vi "Remove vims from files in directory.vi"(8 "error in (no error)":errorcluster, 11 "Folder Path":path) -> (0 "error out":errorcluster)   [LabVIEW 2020]
uses:
  <vilib>/Utility/miscctls.llb/LVMapReplaceAction.ctl
  <vilib>/Utility/traverseref.llb/TRef TravTarget.ctl
  6b92614a-126e-4e2c-8477-dc2805cc9e45.vi
  c56adb90-e54b-4597-b7fa-d326b7dff2e6.vi
  <vilib>/Utility/traverseref.llb/VI Scripting - Traverse.lvlib
panel:
  out "Deleting .vim from disk":path
  out "Disconnecting .vim from library":path
  out "Scanning VI...":path
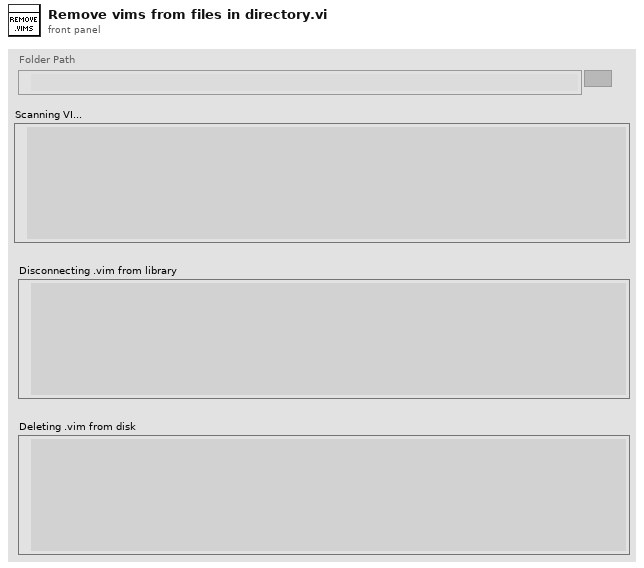
[diagram p1: front panel]
types:
  T1 = enum32{"Invalid", "Standard", "Closed", "Hidden", "Minimized", "Maximized"}
  T2 = typedef "LVMapReplaceAction.ctl" = enum32{"Modify Entry only if found", "Add or Modify Entry", "Delete Entry"}
  T3 = typedef "TRef TravTarget.ctl" = enum16{"FP", "BD", "Other"}
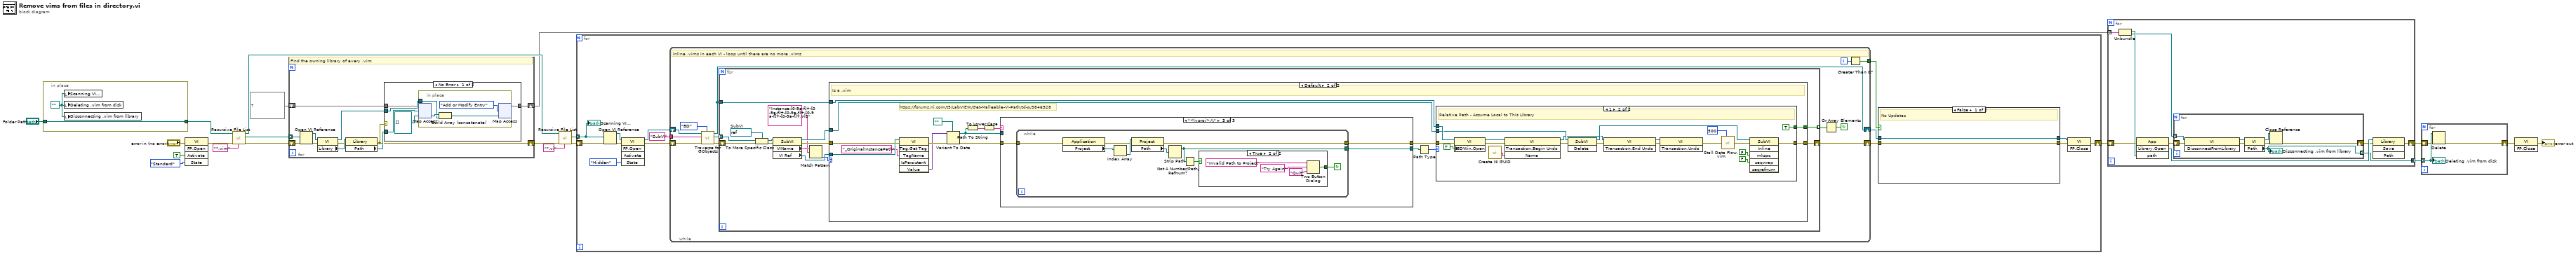
[diagram p0: block diagram]
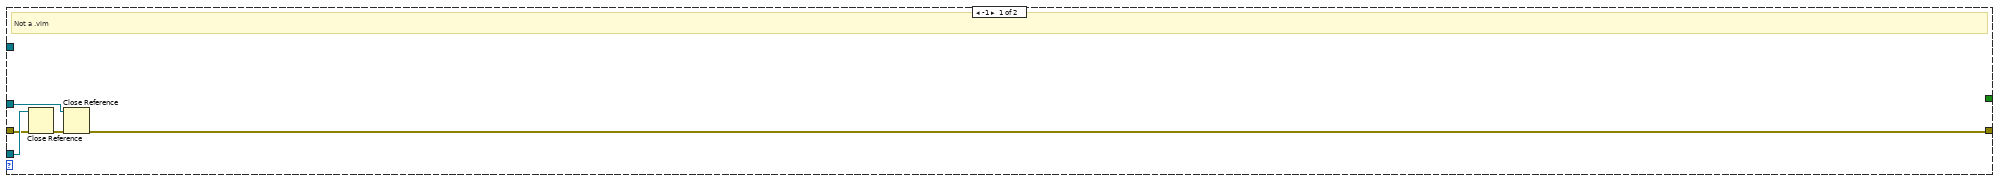
[diagram p2: hidden frame]
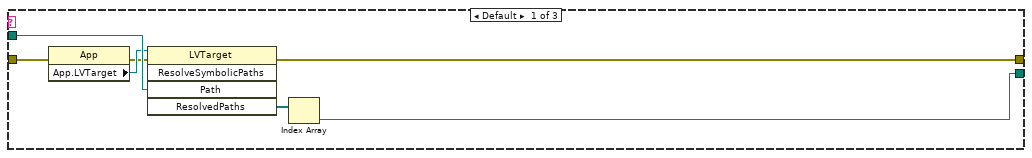
[diagram p3: hidden frame]
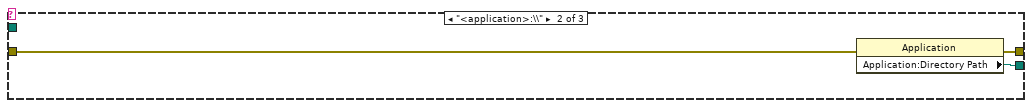
[diagram p4: hidden frame]
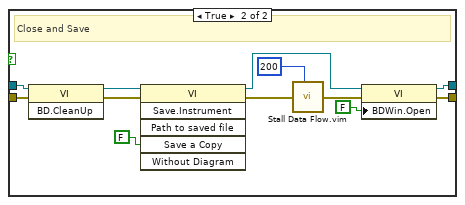
[diagram p7: hidden frame]
diagram:
  n1 = in-place {
    in-place-border: [w22] -> w7
    in-place-border: "Folder Path" -> [w22]
    w23 = path "" ("Scanning VI...")
    n2 = local write "Scanning VI..."(w23) -> ()
    n3 = local write "Deleting .vim from disk"(w23) -> ()
    n4 = local write "Disconnecting .vim from library"(w23) -> ()
  }
  n5 = invoke class="VI" method="FP.Open"(error in="error in (no error)", "Activate"=TRUE ("Activate?"), "State"=T1."Standard") -> (error out=w4:errorcluster)  [unwired: 2 in, 4 out]
  n6 = call <vilib>:"Recursive File List.vi"("pattern"="*.vim", "error in (no error)"=w4, "Folder Path"=w7) -> ("error out"=w19:errorcluster, "All Files in Dir"=w20:path[], "dup Folder Path"=w15:path)  [unwired: 4 in, 2 out]
  n7 = for {
    tunnel: w20 -> [w31] mode=indexing
    shift-right: [w29] -> w11
    shift-left: map{path, refnum<vi>[]} {} ("Size: 0") -> [w28]
    shift-right: [w24] -> w17
    shift-left: w19 -> [w34]
    # "Find the owning library of every .vim"
    n8 = Open VI Reference(vi path=w31, error in (no error)=w34) -> (vi reference=w33:refnum<vi>, error out=w32:errorcluster)  [unwired: 4 in]
    n9 = property class="VI"(reference=w33, error in=w32) -> (reference out=w30:refnum<vi>, error out=w26:errorcluster, "Library"=w27:refnum<vi>)
    n10 = property class="Library"(reference=w27, error in=w26) -> (error out=w24:errorcluster, "Path"=w25:path)  [unwired: 1 out]
    n11 = case shown="No Error" w24 {
      tunnel: w30 -> [w39 _]
      tunnel: [w37 w44] -> w29
      tunnel: w28 -> [w36 w44]
      tunnel: w25 -> [w35 _]
      frame No Error {
        n12 = in-place {
          in-place-border: w39 -> [w41]
          n13 = in-place-map #1(w36, w35, refnum<vi>[] []) -> (w43:refnum<vi>[])  [unwired: 1 out]
          n14 = Build Array (concatenate)(w43, w41) -> (w40:refnum<vi>[])
          n15 = in-place-map #1(w40, LVMapReplaceAction."Add or Modify Entry" ("action")) -> (w37:map{path, refnum<vi>[]})  [unwired: 2 out]
        }
      }
      frame Error {
      }
    }
  }
  n16 = call <vilib>:"Recursive File List.vi"("pattern"="*.vi", "error in (no error)"=w17, "Folder Path"=w15) -> ("error out"=w14:errorcluster, "All Files in Dir"=w13:path[])  [unwired: 4 in, 3 out]
  n17 = for {
    shift-right: [w54] -> w12
    shift-left: w14 -> [w53]
    tunnel: w13 -> [w51] mode=indexing
    n18 = Open VI Reference(vi path=w51, error in (no error)=w53) -> (vi reference=w45:refnum<vi>, error out=w52:errorcluster)  [unwired: 4 in]
    n19 = invoke class="VI" method="FP.Open"(reference=w45, error in=w52, "State"=T1."Hidden") -> (reference out=w55:refnum<vi>, error out=w50:errorcluster)  [unwired: 2 in, 3 out]
    n20 = while {
      shift-right: [w67] -> w48
      shift-left: w55 -> [w68]
      shift-right: [w69] -> w57
      shift-left: w50 -> [w66]
      tunnel: [w60] -> w49
      tunnel: "SubVI" ("Class Name") -> [w59]
      i -> [w61]
      stop <- w62 continue-if-true
      # "Inline .vims in each VI - loop until there are no more .vims"
      n21 = call <vilib>:"Traverse for GObjects.vi"("Traverse Target"=TRef_TravTarget."BD", "error in (no error)"=w66, "Class Name"=w59, "VI Refnum"=w68) -> ("error out"=w65:errorcluster, "References"=w63:refnum<vi>[], "dup VI Refnum"=w67:refnum<vi>)  [unwired: 4 in, 1 out]
      n22 = for {
        shift-right: [w78] -> w69
        shift-left: w65 -> [w84]
        tunnel: w63 -> [w83] mode=indexing
        tunnel: w67 -> [w77]
        tunnel: [w76] -> w70 mode=indexing
        w82 = refnum<vi> refnum  # SubVI
        n23 = To More Specific Class(target class=w82, reference=w83, error in=w84) -> (specific class reference=w81:refnum<vi>, error out=w80:errorcluster)
        n24 = property class="SubVI"(reference=w81, error in=w80) -> (reference out=w72:refnum<vi>, error out=w75:errorcluster, "VIName"=w79:string, "VI Ref"=w73:refnum<vi>)
        n25 = Match Pattern(string=w79, regular expression="Instance:[0-9a-f]+-[0-9a-f]+-[0-9a-f]+-[0-9a-f]+-[0-9a-f]+.vi$") -> (offset past match=w74:i32)  [unwired: 1 in, 3 out]
        n26 = case shown="Default" w74 {
          tunnel: [w89 w106] -> w78
          tunnel: w73 -> [w87 w98]
          tunnel: w77 -> [_ w105]
          tunnel: [_ w104] -> w76
          tunnel: w75 -> [w85 w99]
          tunnel: w72 -> [w88 w103]
          frame -1 {
            # "Not a .vim"
            n27 = Close Reference(reference=w87, error in (no error)=w85) -> (error out=w86:errorcluster)
            n28 = Close Reference(reference=w88, error in (no error)=w86) -> (error out=w89:errorcluster)
          }
          frame Default {
            # "https://forums.ni.com/t5/LabVIEW/Get-Malleable-VI-Path/td-p/3846528"
            # "Is a .vim"
            n29 = invoke class="VI" method="Tag.Get Tag"(reference=w98, error in=w99, "TagName"="_OriginalInstancePath" ("Tag Name")) -> (error out=w102:errorcluster, "Value"=w101:variant)  [unwired: 3 in, 4 out]
            n30 = Variant To Data(error in=w102, type=path "", Variant=w101) -> (data=w94:path, error out=w97:errorcluster)
            n31 = Path To String(path=w94) -> (string=w90:string)
            n32 = To Lower Case(string=w90) -> (all lower case string=w91:string)
            n33 = case shown="\"<lvproj>:\\\\\"" w91 {
              tunnel: w94 -> [w110 _ _]
              tunnel: [w113 w116 w117] -> w93
              tunnel: [w112 w115 w119] -> w95
              tunnel: w97 -> [w111 w114 w118]
              frame Default {
                n34 = property class="App"(error in=w111) -> (error out=w108:errorcluster, "App.LVTarget"=w109:refnum<vi>)  [unwired: 1 in, 1 out]
                n35 = invoke class="LVTarget" method="ResolveSymbolicPaths"(reference=w109, error in=w108, "Path"=w110) -> (error out=w112:errorcluster, "ResolvedPaths"=w107:path[])  [unwired: 2 in, 3 out]
                n36 = Index Array(array=w107) -> (element=w113:path)  [unwired: 1 in]
              }
              frame "<application>:\\" {
                n37 = property class="Application"(error in=w114) -> (error out=w115:errorcluster, "Application:Directory Path"=w116:path)  [unwired: 1 in, 1 out]
              }
              frame "<lvproj>:\\" {
                n38 = while {
                  tunnel: [w125] -> w119
                  tunnel: w118 -> [w124]
                  tunnel: [w121] -> w117
                  stop <- w120 continue-if-true
                  n39 = property class="Application"(error in=w124) -> (error out=w126:errorcluster, "Project"=w128:refnum<vi>[])  [unwired: 1 in, 1 out]
                  n40 = Index Array(array=w128) -> (element=w127:refnum<vi>)  [unwired: 1 in]
                  n41 = property class="Project"(reference=w127, error in=w126) -> (error out=w125:errorcluster, "Path"=w123:path)  [unwired: 1 out]
                  n42 = Strip Path(path=w123) -> (stripped path=w121:path)  [unwired: 1 out]
                  n43 = Not A Number/Path/Refnum?(number/path/refnum=w121) -> (NaN/Path/Refnum?=w122:bool)
                  n44 = case shown="True" w122 {
                    tunnel: [_ w129] -> w120
                    frame False {
                    }
                    frame True {
                      n45 = Two Button Dialog(message="Invalid Path to Project", 1:"Quit" ("F button name (\"Cancel\")"), 2:"Try Again" ("T button name (\"OK\")")) -> (T button?=w129:bool)
                    }
                  }
                }
              }
            }
            n46 = Path Type(1:w93) -> (0:w92:i16)
            n47 = case shown="1" w92 {
              tunnel: w105 -> [_ w153]
              tunnel: [w133 w152] -> w106
              tunnel: [_ TRUE] -> w104
              tunnel: w95 -> [w133 w150]
              tunnel: w103 -> [_ w149]
              frame Default {
              }
              frame 1 {
                # "Relative Path - Assume Local to This Library"
                n48 = property class="VI"(reference=w153, error in=w150, "BDWin.Open"=TRUE ("Block Diagram Window:Open")) -> (reference out=w141:refnum<vi>, error out=w143:errorcluster)
                n49 = call <vilib>:"Create NI GUID.vi"() -> ("NI GUID"=w134:string)
                n50 = invoke class="VI" method="Transaction.Begin Undo"(reference=w141, error in=w143, "Name"=w134) -> (reference out=w137:refnum<vi>, error out=w135:errorcluster)  [unwired: 1 in, 2 out]
                n51 = invoke class="SubVI" method="Delete"(reference=w149, error in=w135) -> (reference out=w144:refnum<vi>, error out=w136:errorcluster)  [unwired: 1 in, 1 out]
                n52 = invoke class="VI" method="Transaction.End Undo"(reference=w137, error in=w136) -> (reference out=w138:refnum<vi>, error out=w139:errorcluster)  [unwired: 1 in, 1 out]
                n53 = invoke class="VI" method="Transaction.Undo"(reference=w138, error in=w139) -> (error out=w140:errorcluster)  [unwired: 1 in, 2 out]
                n54 = call "Stall Data Flow.vim"("value in"=w140, "milliseconds to wait"=u32 500) -> ("value out"=w146:errorcluster)  [unwired: 1 out]
                n55 = invoke class="SubVI" method="Inline"(reference=w144, error in=w146, "mkspc"=FALSE ("Make Space in Block Diagram"), "seqwrap"=FALSE ("Wrap in Sequence")) -> (error out=w152:errorcluster)  [unwired: 2 in, 5 out]
              }
            }
          }
        }
      }
      n56 = Or Array Elements(Boolean array=w70) -> (logical OR=w62:bool)
      n57 = Greater Than 0?(x=w61) -> (x > 0?=w60:bool)
    }
    n58 = case shown="False" w49 {
      tunnel: w48 -> [w154 w167]
      tunnel: w57 -> [w155 w166]
      tunnel: [w155 w160] -> w56
      tunnel: [w154 w156] -> w47
      frame False {
        # "No Updates"
      }
      frame True {
        # "Close and Save"
        n59 = invoke class="VI" method="BD.CleanUp"(reference=w167, error in=w166) -> (reference out=w164:refnum<vi>, error out=w163:errorcluster)  [unwired: 1 in, 1 out]
        n60 = invoke class="VI" method="Save.Instrument"(reference=w164, error in=w163, "Save a Copy"=FALSE) -> (reference out=w161:refnum<vi>, error out=w162:errorcluster)  [unwired: 3 in, 4 out]
        n61 = call "Stall Data Flow.vim"("value in"=w162, "milliseconds to wait"=u32 200) -> ("value out"=w158:errorcluster)  [unwired: 1 out]
        n62 = property class="VI"(reference=w161, error in=w158, "BDWin.Open"=FALSE ("Block Diagram Window:Open")) -> (reference out=w156:refnum<vi>, error out=w160:errorcluster)
      }
    }
    n63 = invoke class="VI" method="FP.Close"(reference=w47, error in=w56) -> (error out=w54:errorcluster)  [unwired: 1 in, 2 out]
    "Scanning VI..." <- w51
  }
  n64 = for {
    shift-right: [w169] -> w9
    shift-left: w12 -> [w175]
    tunnel: w11 -> [w176] mode=indexing
    tunnel: [w168] -> w10 mode=concatenating
    n65 = Unbundle(w176) -> ("Library"=w174:path, w172:refnum<vi>[])
    n66 = invoke class="App" method="Library.Open"(error in=w175, "path"=w174) -> (error out=w173:errorcluster, "Open Library"=w171:refnum<vi>)  [unwired: 2 in, 2 out]
    n67 = for {
      shift-right: [w179] -> w170
      shift-left: w173 -> [w183]
      tunnel: w172 -> [w184] mode=indexing
      tunnel: [w177] -> w168 mode=indexing
      n68 = invoke class="VI" method="DisconnectFromLibrary"(reference=w184, error in=w183) -> (reference out=w181:refnum<vi>, error out=w182:errorcluster)  [unwired: 1 in, 1 out]
      n69 = property class="VI"(reference=w181, error in=w182) -> (reference out=w178:refnum<vi>, error out=w180:errorcluster, "Path"=w177:path)
      "Disconnecting .vim from library" <- w177
      n70 = Close Reference(reference=w178, error in (no error)=w180) -> (error out=w179:errorcluster)
    }
    n71 = invoke class="Library" method="Save"(reference=w171, error in=w170) -> (error out=w169:errorcluster)  [unwired: 2 in, 3 out]
  }
  n72 = for {
    tunnel: w10 -> [w185] mode=indexing
    shift-right: [w186] -> w8
    shift-left: w9 -> [w187]
    n73 = Delete(path (use dialog)=w185, error in=w187) -> (error out=w186:errorcluster)  [unwired: 3 in, 2 out]
    "Deleting .vim from disk" <- w185
  }
  n74 = invoke class="VI" method="FP.Close"(error in=w8) -> (error out=→"error out":errorcluster)  [unwired: 2 in, 2 out]
